vi "Delete Object.vi"(6 "Auth device data":T2, 7 "Version ID":string, 8 "error in (no error)":errorcluster, 9 "Bucket":string, 10 "Object path":string) -> (0 "error out":errorcluster, 3 "Versioning Data":T1)   [LabVIEW 2011, in "LV Interface for Amazon S3.lvlib"]
doc: "The operation <B>removes the null version</B> (if there is one) <B>of an object and inserts a delete marker</B>, which becomes the latest version of the object. If there isn't a null version, Amazon S3 does not remove any objects."
uses:
  LV Interface for Amazon S3.lvlib
  Typedefs/AMZ_S3_Auth Device Data.ctl
  Typedefs/AMZ_S3_API_Delete Object with Versioning Result.ctl
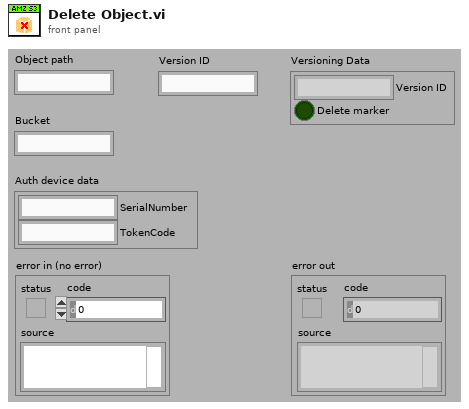
[diagram p1: front panel]
types:
  T1 = typedef "LV Interface for Amazon S3.lvlib/AMZ_S3_API_Delete Object with Versioning Result.ctl" = cluster{"Version ID":string, "Delete marker":bool}
  T2 = typedef "LV Interface for Amazon S3.lvlib/AMZ_S3_Auth Device Data.ctl" = cluster{"SerialNumber":string, "TokenCode":string}
  T3 = typedef "LV Interface for Amazon S3.lvlib/AMZ_S3_HTTP Header-Value pair.ctl" = cluster{"Header":string, "Value":string}
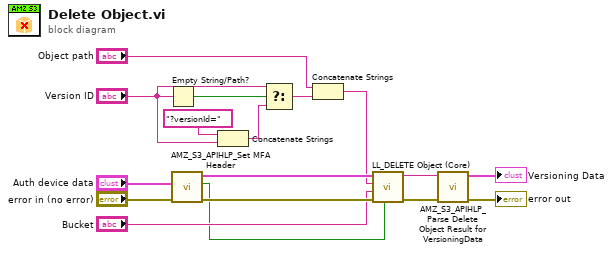
[diagram p0: block diagram]
diagram:
  n1 = Empty String/Path?(string/path="Version ID") -> (empty?=w15:bool)
  n2 = call "AMZ_S3_APIHLP_Set MFA Header.vi"("error in (no error)"="error in (no error)", "Auth device data"="Auth device data") -> ("error out"=w9:errorcluster, "Header set?"=w1:bool, "HTTP Headers"=w8:T3[])  [unwired: 7 in]
  n3 = Concatenate Strings("?versionId=", "Version ID") -> (w12:string)
  n4 = Select(t="Version ID", s=w15, f=w12) -> (s? t:f=w11:string)
  n5 = Concatenate Strings("Object path", w11) -> (w7:string)
  n6 = call "LL_DELETE Object (Core).vi"("Use HTTPS?"=w1, "error in (no error)"=w9, "Bucket"="Bucket", "Path and query string"=w7, "Headers"=w8) -> ("error out"=w5:errorcluster, "Response header"=w4:string)  [unwired: 3 in, 2 out]
  n7 = call "AMZ_S3_APIHLP_Parse Delete Object Result for VersioningData.vi"("error in (no error)"=w5, "Response header"=w4) -> ("error out"=→"error out":errorcluster, "Versioning Data"=→"Versioning Data":T1)  [unwired: 8 in]
